vi "XML.Sequences.LoadIntoArray.vi"(8 "error in":errorcluster, 10 "XML file path":path=path "C:/Projects/TM-OS/trunk/Design/XML_HW_config2.xml") -> (0 "error out":errorcluster, 2 "sequences array":T1[](array[typedef]))   [LabVIEW 2019, in "Tools.lvlib"]
uses:
  Tools.lvlib
  <vilib>/xml/NI_XML.lvlib
  Modules/Sequences_Management/Gui/Sequences_Management.Gui.Product.ctl
  <vilib>/xml/Close Reference(Node).vi
  <vilib>/xml/Load XML File.vi
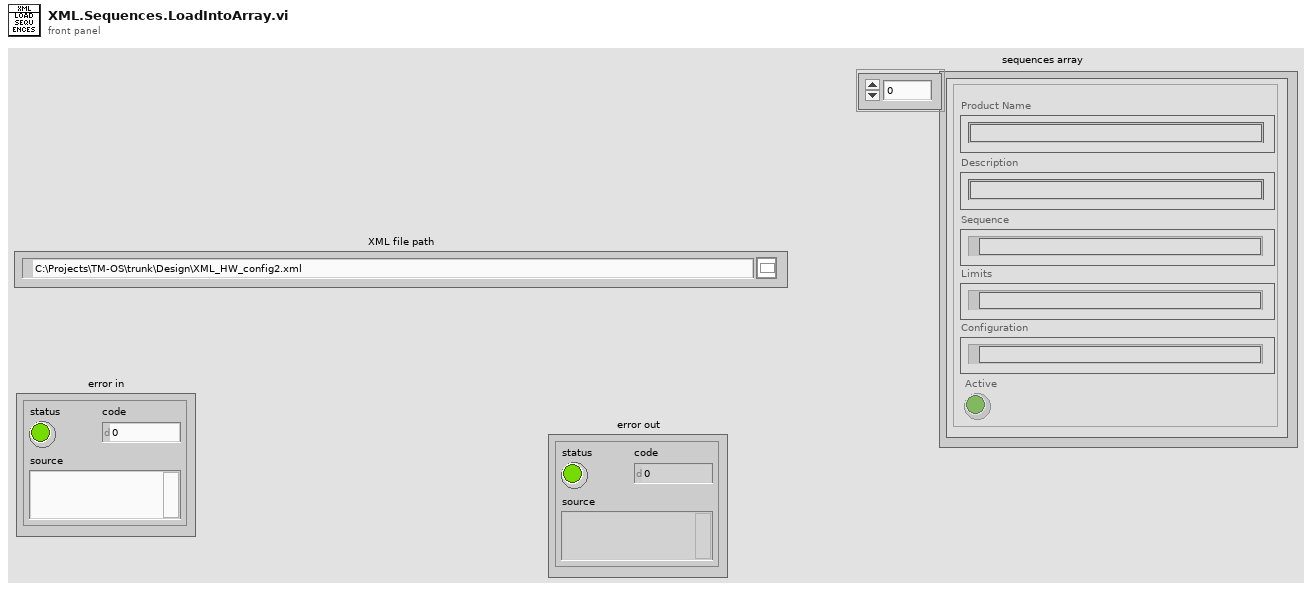
[diagram p1: front panel]
types:
  T1 = typedef "Sequences_Management.Gui.Product.ctl" = cluster{"Product Name":string, "Description":string, "Sequence":path, "Limits":path, "Configuration":path, "Active":bool}
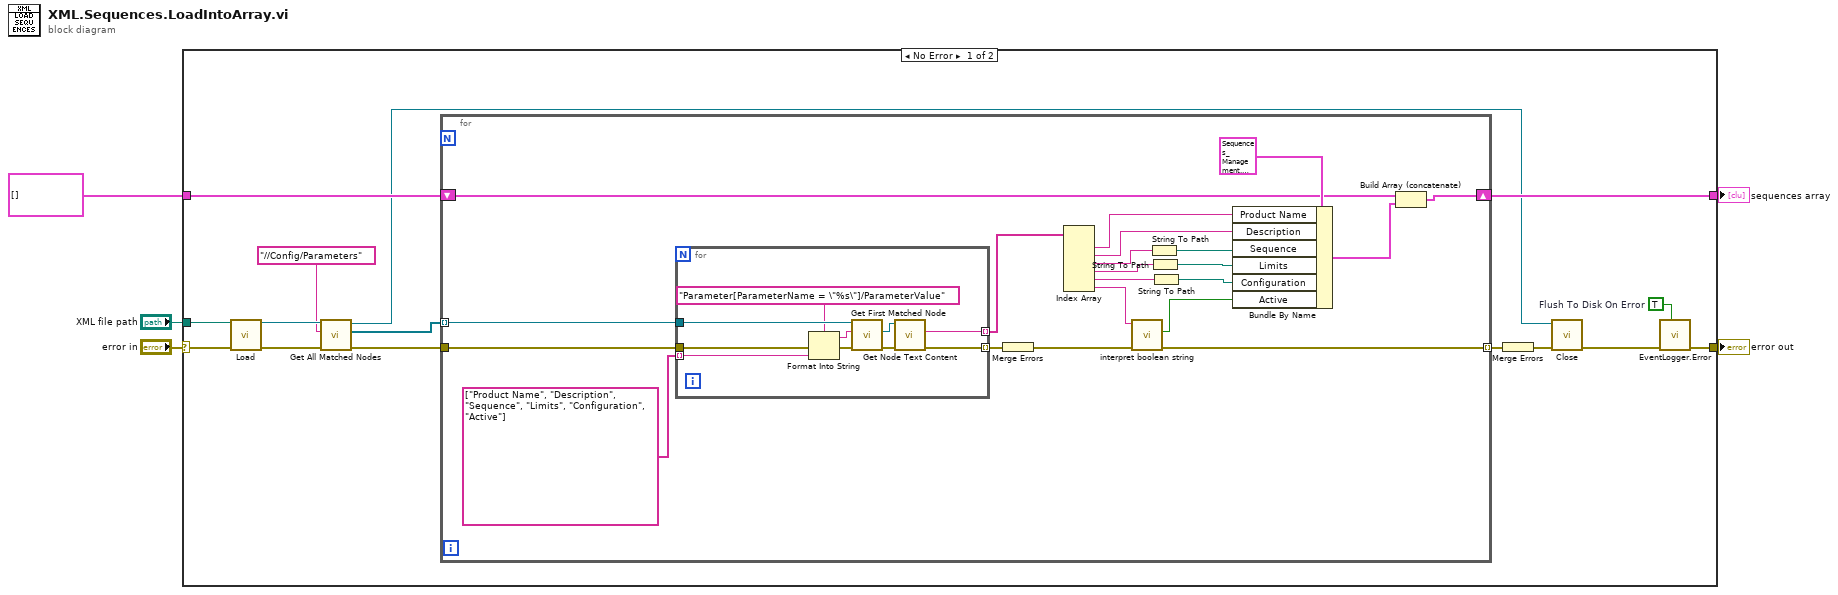
[diagram p0: block diagram]
diagram:
  n1 = case shown="No Error" "error in" {
    selector: "error in" -> [w17 w53]
    tunnel: [w7 w53] -> w5
    tunnel: "XML file path" -> [w18 _]
    tunnel: T1[] [] -> [w19 w52]
    tunnel: [w11 w52] -> w1
    frame No Error {
      w6 = TRUE  # Flush To Disk On Error
      n2 = call-poly <vilib>:"Load.vi"("path to XML document"=w18, "error in (no error)"=w17) -> ("DOM document out"=w15:refnum<k20>, "error out"=w16:errorcluster)  [unwired: 11 in, 1 out]
      n3 = call <vilib>:"Get All Matched Nodes.vi"("error in (no error)"=w16, "XPath expression"="//Config/Parameters", "node in"=w15) -> ("error out"=w14:errorcluster, "node result array"=w13:refnum<k20>[], "node out"=w9:refnum<k20>)  [unwired: 6 in]
      n4 = for {
        shift-right: [w31] -> w11
        shift-left: w19 -> [w33]
        tunnel: w13 -> [w41] mode=indexing
        tunnel: w14 -> [w23]
        tunnel: [w21] -> w20 mode=indexing
        n5 = for {
          tunnel: w41 -> [w51]
          tunnel: string[] ["Product Name", "Description", "Sequence", "Limits", "Configuration", "Active"] -> [w45] mode=indexing
          tunnel: [w44] -> w38 mode=indexing
          tunnel: [w43] -> w24 mode=indexing
          tunnel: w23 -> [w42]
          n6 = Format Into String(format string="Parameter[ParameterName = \"%s\"]/ParameterValue" ("XPath expression"), error in=w42, w45) -> (resulting string=w49:string, error out=w47:errorcluster)  [unwired: 1 in]
          n7 = call <vilib>:"Get First Matched Node.vi"("error in (no error)"=w47, "XPath expression"=w49, "node in"=w51) -> ("error out"=w46:errorcluster, "node result"=w48:refnum<k20>)  [unwired: 6 in, 1 out]
          n8 = call <vilib>:"Get Node Text Content.vi"("error in (no error)"=w46, "node in"=w48) -> ("error out"=w43:errorcluster, "node text"=w44:string)  [unwired: 7 in, 1 out]
        }
        n9 = Merge Errors(w24) -> (w22:errorcluster)
        n10 = Index Array(array=w38) -> (element #1=w37:string, element #2=w30:string, element #3=w29:string, element #4=w28:string, element #5=w27:string, element #6=w26:string)  [unwired: 6 in]
        n11 = call "interpret boolean string.vi"("error in (no error)"=w22, "string"=w26) -> ("error out"=w21:errorcluster, "value"=w25:bool)  [unwired: 8 in]
        n12 = String To Path(string=w29) -> (path=w36:path)
        n13 = String To Path(string=w28) -> (path=w35:path)
        n14 = String To Path(string=w27) -> (path=w34:path)
        n15 = Bundle By Name(cluster=T1 {"Product Name"="", "Description"="", "Sequence"=path "", "Limits"=path "", "Configuration"=path "", "Active"=FALSE} ("Cluster"), "Product Name"=w37, "Description"=w30, "Sequence"=w36, "Limits"=w35, "Configuration"=w34, "Active"=w25) -> (w32:T1)
        n16 = Build Array (concatenate)(w33, w32) -> (w31:T1[])
      }
      n17 = Merge Errors(w20) -> (w10:errorcluster)
      n18 = call-poly <vilib>:"Close.vi"("error in (no error)"=w10, "node"=w9) -> ("error out"=w8:errorcluster)  [unwired: 7 in]
      n19 = call "EventLogger.Error.vi"("Flush To Disk On Error"=w6, "error in"=w8) -> ("error out"=w7:errorcluster)  [unwired: 9 in]
    }
    frame Error {
    }
  }
  "error out" <- w5
  "sequences array" <- w1
